vi "Test Framework.vi"(7 "Write (F)":bool, 10 "Test Framework (Unknown)":T1) -> (2 "Test Framework out":T1)   [LabVIEW 2017, in "Transparent Assertions.lvlib" / "Configuration.lvlib" / "Global Configuration.lvlib"]
doc: "Gets or sets the test framework used for assertions. If the framework is set to <B>Unknown</B>, the library will automatically detect an appropriate test framework based on the application context."
uses:
  Global Configuration.lvlib
  Frameworks/Test Framework.ctl
  Frameworks/Frameworks.lvlib
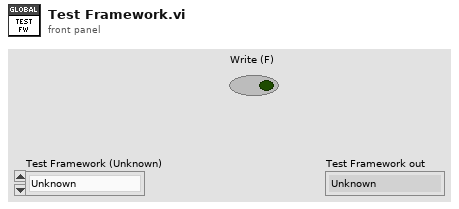
[diagram p1: front panel]
types:
  T1 = typedef "Transparent Assertions.lvlib/Frameworks.lvlib/Test Framework.ctl" = enum16{"Unknown", "LVUnit", "Caraya"}
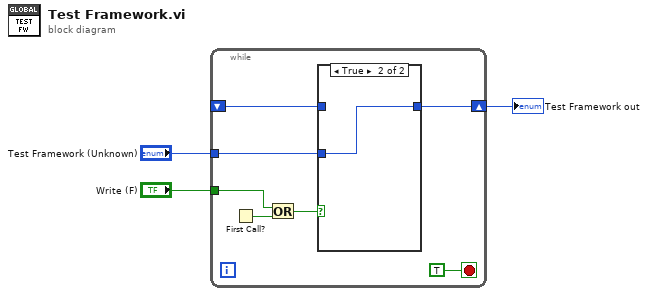
[diagram p0: block diagram]
diagram:
  n1 = while {
    shift-right: [w5] -> w3
    shift-left: _ -> [w6]
    tunnel: "Write (F)" -> [w8]
    tunnel: "Test Framework (Unknown)" -> [w4]
    stop <- TRUE stop-if-true
    n2 = First Call?() -> (First Call?: T/F=w9:bool)
    n3 = Or(x=w8, y=w9) -> (x .or. y?=w7:bool)
    n4 = case shown="True" w7 {
      tunnel: w6 -> [w11 _]
      tunnel: [w11 w12] -> w5
      tunnel: w4 -> [_ w12]
      frame False {
      }
      frame True {
      }
    }
  }
  "Test Framework out" <- w3
